vi "VI_Dynamic Load by Ref.vi"(6 "Auto Dispose Ref":bool, 7 "FrontPanel(close)":T2(ring)=enum."Closed", 8 "error in":errorcluster, 9 "CtrlValue":variant, 10 "CtrlName":string, 11 "Static vi reference in":refnum<vi>) -> (0 "错误输出":errorcluster caption="error out", 2 "Exec.State":T1(ring), 3 "Dynamic vi reference out":refnum<vi>)   [LabVIEW 2016]
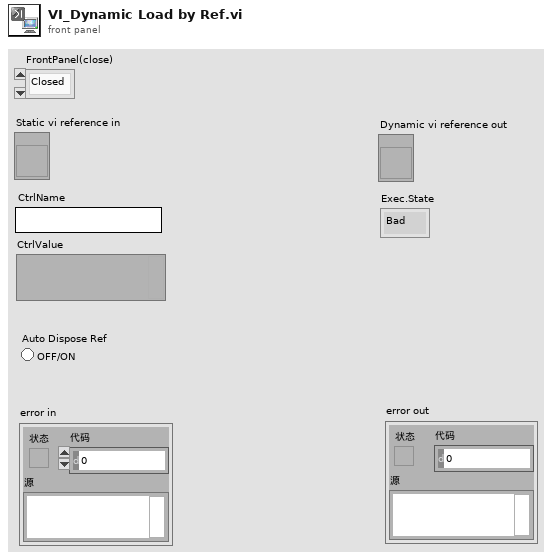
[diagram p1: front panel]
types:
  T1 = enum32{"Bad", "Idle", "Run top level", "Running"}
  T2 = enum32{"Invalid", "Standard", "Closed", "Hidden", "Minimized", "Maximized"}
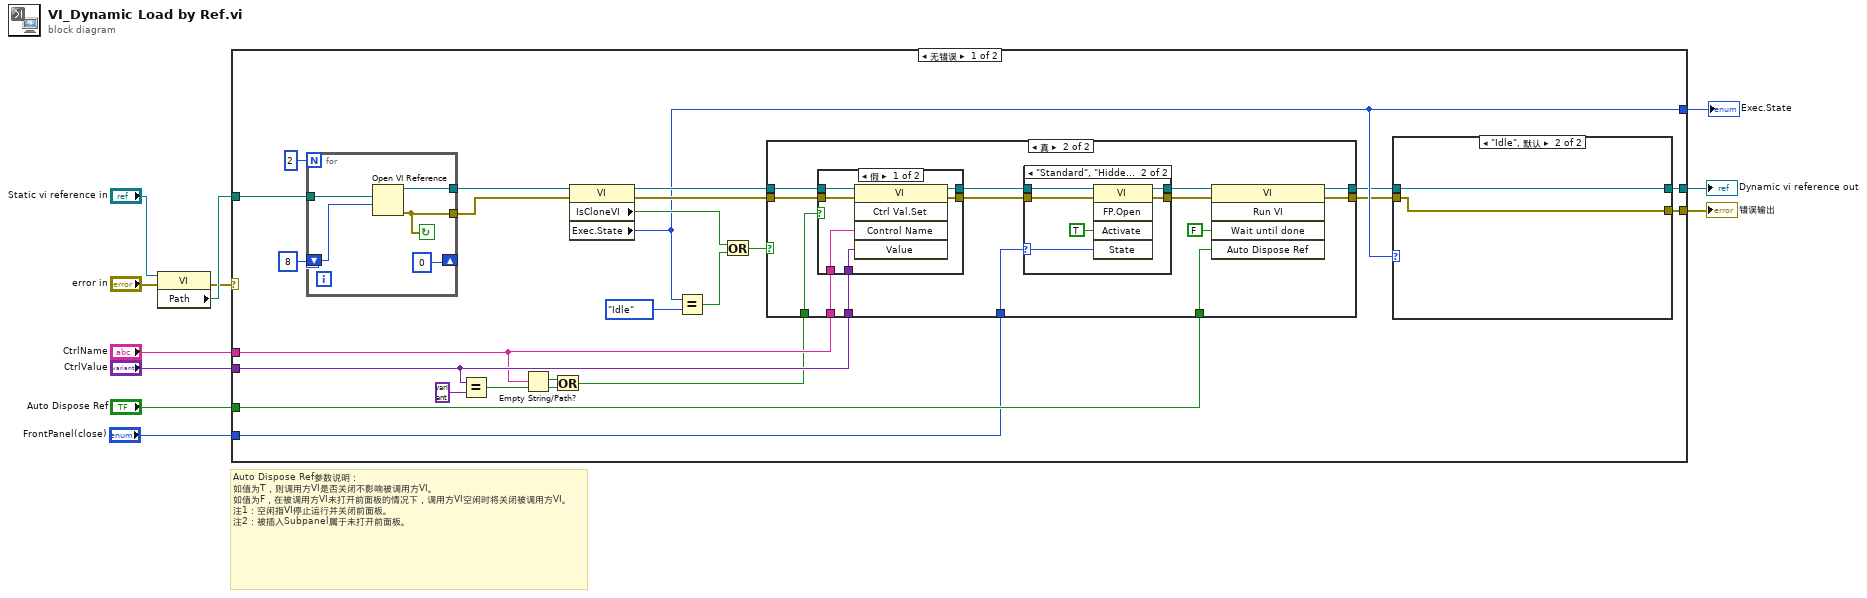
[diagram p0: block diagram]
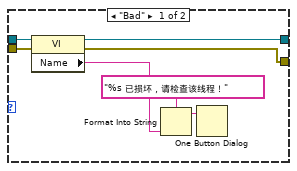
[diagram p2: hidden frame]
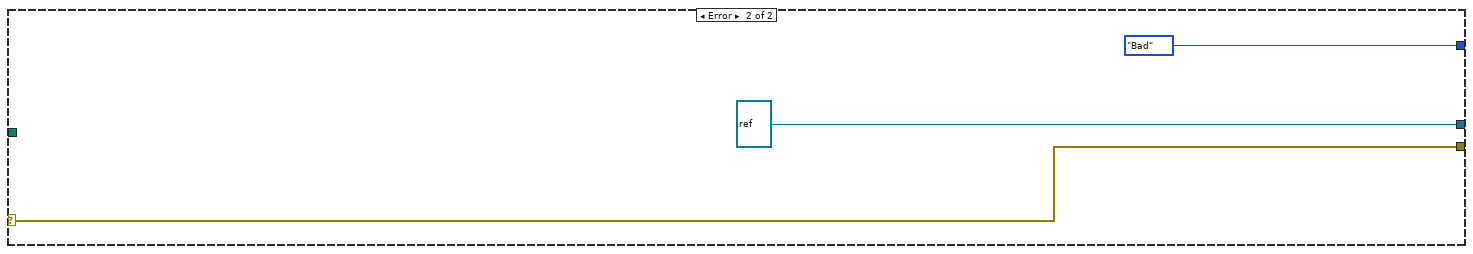
[diagram p6: hidden frame]
diagram:
  # "Auto Dispose Ref参数说明：\n如值为T，则调用方VI是否关闭不影响被调用方VI。\n如值为F，在被调用方VI未打开前面板的情况下，调用方VI空闲时将关闭被调用方VI。\n注1：空闲指VI停止运行并关闭前面板。\n注2：被插入Subpanel属于未打开前面板。"
  n1 = property class="VI"(reference="Static vi reference in", error in="error in") -> (error out=w3:errorcluster, "Path"=w5:path)  [unwired: 1 out]
  n2 = case shown="无错误" w3 {
    selector: w3 -> [_ w83]
    tunnel: [w13 refnum<vi> refnum ("vi reference")] -> w11
    tunnel: [w12 w83] -> w10
    tunnel: "Auto Dispose Ref" -> [w27 _]
    tunnel: "CtrlName" -> [w24 _]
    tunnel: "CtrlValue" -> [w26 _]
    tunnel: w5 -> [w20 _]
    tunnel: "FrontPanel(close)" -> [w19 _]
    tunnel: [w16 T1."Bad" ("Exec.State")] -> w1
    frame No Error {
      n3 = for {
        N: 2 -> [_]
        tunnel: w20 -> [w49]
        shift-right: [0 ("选项")] -> _
        shift-left: 8 ("选项") -> [w48]
        tunnel: [w46] -> w17
        tunnel: [w45] -> w18
        stop <- w46 continue-if-true
        n4 = Open VI Reference(vi path=w49, options=w48) -> (vi reference=w45:refnum<vi>, error out=w46:errorcluster)  [unwired: 4 in]
      }
      n5 = Equal?(x=w26, y=variant) -> (x = y?=w22:bool)
      n6 = Empty String/Path?(string/path=w24) -> (empty?=w23:bool)
      n7 = Or(x=w23, y=w22) -> (x .or. y?=w21:bool)
      n8 = property class="VI"(reference=w18, error in=w17) -> (reference out=w35:refnum<vi>, error out=w34:errorcluster, "IsCloneVI"=w30:bool, "Exec.State"=w16:T1)
      n9 = Equal?(x=w16, y=T1."Idle") -> (x = y?=w29:bool)
      n10 = Or(x=w30, y=w29) -> (x .or. y?=w28:bool)
      n11 = case shown="真" w28 {
        tunnel: w35 -> [w51 w61]
        tunnel: [w51 w65] -> w15
        tunnel: w34 -> [w50 w60]
        tunnel: [w50 w64] -> w14
        tunnel: w27 -> [_ w62]
        tunnel: w24 -> [_ w59]
        tunnel: w26 -> [_ w58]
        tunnel: w21 -> [_ w57]
        tunnel: w19 -> [_ w52]
        frame False {
        }
        frame True {
          n12 = case shown="假" w57 {
            tunnel: w61 -> [w79 w81]
            tunnel: [w78 w81] -> w56
            tunnel: w60 -> [w77 w80]
            tunnel: [w76 w80] -> w55
            tunnel: w59 -> [w75 _]
            tunnel: w58 -> [w74 _]
            frame False {
              n13 = invoke class="VI" method="Ctrl Val.Set"(reference=w79, error in=w77, "Control Name"=w75, "Value"=w74) -> (reference out=w78:refnum<vi>, error out=w76:errorcluster)  [unwired: 1 in, 3 out]
            }
            frame True {
            }
          }
          n14 = case shown="\"Standard\", \"Hidden\"..\"Maximized\"" w52 {
            selector: w52 -> [_ w68]
            tunnel: w56 -> [w67 w73]
            tunnel: w55 -> [w66 w72]
            tunnel: [w67 w71] -> w54
            tunnel: [w66 w70] -> w53
            frame "Invalid", Default {
            }
            frame "Standard", "Hidden".."Maximized" {
              n15 = invoke class="VI" method="FP.Open"(reference=w73, error in=w72, "Activate"=TRUE ("激活？"), "State"=w68) -> (reference out=w71:refnum<vi>, error out=w70:errorcluster)  [unwired: 1 in, 3 out]
            }
          }
          n16 = invoke class="VI" method="Run VI"(reference=w54, error in=w53, "Wait until done"=FALSE ("结束前等待"), "Auto Dispose Ref"=w62) -> (reference out=w65:refnum<vi>, error out=w64:errorcluster)  [unwired: 1 in, 3 out]
        }
      }
      n17 = case shown="\"Idle\", 默认" w16 {
        tunnel: w15 -> [w39 w44]
        tunnel: w14 -> [w40 w43]
        tunnel: [w37 w44] -> w13
        tunnel: [w36 w43] -> w12
        frame "Bad" {
          n18 = property class="VI"(reference=w39, error in=w40) -> (reference out=w37:refnum<vi>, error out=w36:errorcluster, "Name"=w38:string)
          n19 = Format Into String(format string="%s 已损坏，请检查该线程！" ("格式字符串"), w38) -> (resulting string=w42:string)  [unwired: 2 in, 1 out]
          n20 = One Button Dialog(message=w42) -> ()  [unwired: 1 in, 1 out]
        }
        frame "Idle", Default {
        }
      }
    }
    frame Error {
    }
  }
  "Dynamic vi reference out" <- w11
  "错误输出" <- w10
  "Exec.State" <- w1
